vi "Fault Latch Test.vi"(4 "Clear Latch":bool, 5 "Faults":bool[](array[boolean])=[FALSE, FALSE, FALSE, FALSE, FALSE, FALSE, FALSE]) -> (1 "Latched Fault":bool[](array[boolean]))   [LabVIEW 2014]
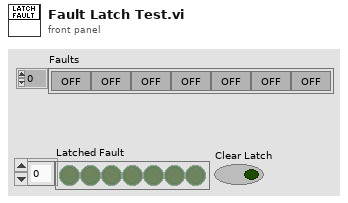
[diagram p1: front panel]
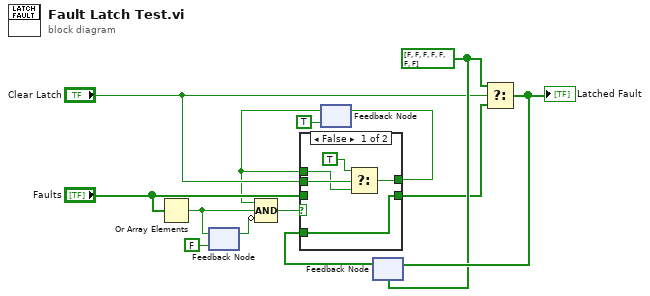
[diagram p0: block diagram]
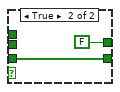
[diagram p2: hidden frame]
diagram:
  w9 = bool[] [FALSE, FALSE, FALSE, FALSE, FALSE, FALSE, FALSE] ("Latched Fault")
  n1 = Or Array Elements(Boolean array="Faults") -> (logical OR=w12:bool)
  n2 = feedback #1(FALSE) -> (w11:bool)
  n3 = feedback-in #1(w12) -> ()
  n4 = feedback #2(TRUE) -> (w1:bool)
  n5 = Compound Arithmetic op=AND(w1, w12, invert w11) -> (w8:bool)
  n6 = feedback #3(w9) -> (w7:bool[])
  n7 = case shown="False" w8 {
    tunnel: w7 -> [w14 _]
    tunnel: [w14 w20] -> w6
    tunnel: "Faults" -> [_ w20]
    tunnel: [w15 FALSE] -> w4
    tunnel: "Clear Latch" -> [w18 _]
    tunnel: w1 -> [w17 _]
    frame False {
      n8 = Select(t=TRUE, s=w18, f=w17) -> (s? t:f=w15:bool)
    }
    frame True {
    }
  }
  n9 = feedback-in #2(w4) -> ()
  n10 = Select(t=w9, s="Clear Latch", f=w6) -> (s? t:f=w10:bool[])
  "Latched Fault" <- w10
  n11 = feedback-in #3(w10) -> ()
